vi "Disconnect.vi"(8 "error in (no error)":errorcluster, 11 "reference in":refnum<class "NS master.lvclass">) -> (0 "error out":errorcluster, 3 "reference out":refnum<class "NS master.lvclass">)   [LabVIEW 2019, in "CommandResponse communication.lvlib" / "NS master.lvclass"]
doc: "Close all network streams to slave"
uses:
  NS master.lvclass
  ITC command.ctl
  ITC response.ctl
  CommandResponse communication.lvlib
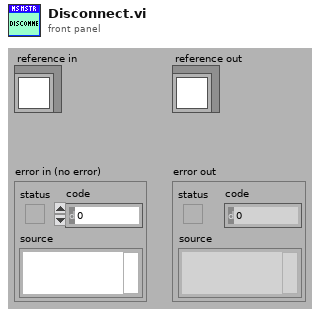
[diagram p1: front panel]
types:
  T1 = typedef "CommandResponse communication.lvlib/NS master.lvclass/ObjectAttributesRef.ctl" = refnum<data-value>
  T2 = typedef "CommandResponse communication.lvlib/NS master.lvclass/ObjectAttributes.ctl" = cluster{"connected":bool, "stop":bool, "ID":string, "command wr":refnum<k21>, "response rd":refnum<k21>, "data rd":refnum<k21>, "slave ip":string, "slave id":string}
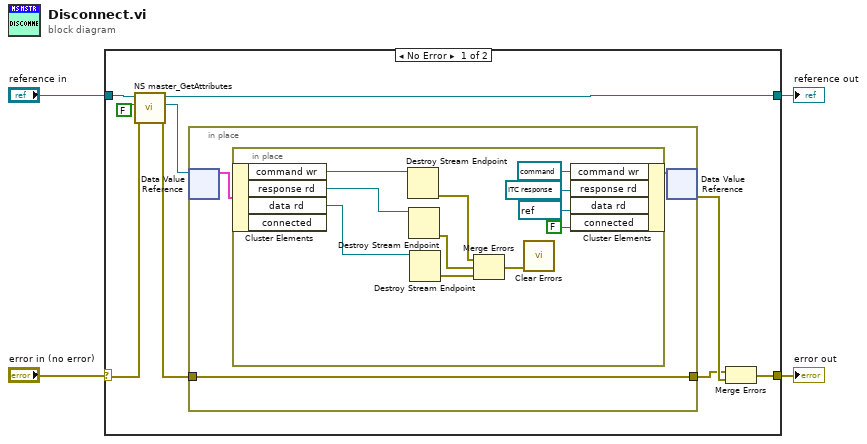
[diagram p0: block diagram]
diagram:
  n1 = case shown="No Error" "error in (no error)" {
    selector: "error in (no error)" -> [w8 w29]
    tunnel: [w13 w29] -> w3
    tunnel: [w6 w28] -> w1
    tunnel: "reference in" -> [w10 w28]
    frame No Error {
      n2 = call "NS master_GetAttributes.vi"("error in (no error)"=w8, "return data? (T)"=FALSE, "reference in"=w10) -> ("error out"=w7:errorcluster, "attributes ref"=w5:T1, "reference out"=w6:refnum<class "NS master.lvclass">)  [unwired: 5 in, 1 out]
      n3 = in-place {
        in-place-border: w7 -> [w14]
        in-place-border: [w14] -> w11
        n4 = in-place-dvr #1(w5) -> (w15:T2)  [unwired: 1 out]
        n5 = in-place {
          n6 = in-place-cluster #2(w15) -> ("command wr"=w27:refnum<k21>, "response rd"=w23:refnum<k21>, "data rd"=w22:refnum<k21>)  [unwired: 1 out]
          n7 = Destroy Stream Endpoint(11:w27) -> (0:w19:errorcluster)  [unwired: 1 in]
          n8 = Destroy Stream Endpoint(11:w23) -> (0:w18:errorcluster)  [unwired: 1 in]
          n9 = Destroy Stream Endpoint(11:w22) -> (0:w20:errorcluster)  [unwired: 1 in]
          n10 = Merge Errors(w19, w18, w20) -> (w17:errorcluster)
          n11 = call <vilib>:"Clear Errors.vi"("error in (no error)"=w17) -> ()  [unwired: 5 in, 2 out]
          n12 = in-place-cluster #2("command wr"=refnum<k21> refnum, "response rd"=refnum<k21> refnum, "data rd"=refnum<k21> refnum, "connected"=FALSE) -> (w16:T2)
        }
        n13 = in-place-dvr #1(w16) -> (w12:errorcluster)  [unwired: 1 out]
      }
      n14 = Merge Errors(w11, w12) -> (w13:errorcluster)
    }
    frame Error {
    }
  }
  "error out" <- w3
  "reference out" <- w1
